vi "FCO_Open232.vi"(10 "port":u32, 11 "VISA resource name":refnum<visa-resource-name> caption="VISA资源名称") -> (0 "错误输出":errorcluster, 3 "status":bool)   [LabVIEW 2017]
uses:
  <vilib>/Instr/_visa.llb/VISA Configure Serial Port (Instr).vi
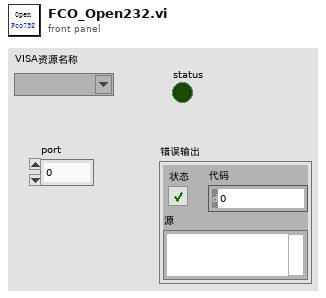
[diagram p1: front panel]
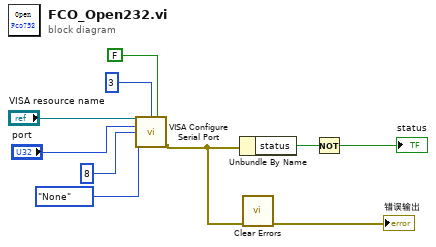
[diagram p0: block diagram]
diagram:
  n1 = call-poly "VISA Configure Serial Port"("VISA resource name"="VISA resource name", "termination char\n(0xA = '\\n' = LF)"=u8 3 ("termination char\n(0xA = '\\n' = LF)"), "Enable Termination\nChar (T)"=FALSE ("Enable Termination\nChar (T)"), "baud rate (9600)"="port", "data bits (8)"=u16 8, "parity (0:none)"=enum16{"None", "Odd", "Even", "Mark", "Space"}."None") -> ("error out"=w5:errorcluster)  [unwired: 4 in, 5 out]
  n2 = Unbundle By Name(w5) -> ("status"=w7:bool)
  n3 = call <vilib>:"Clear Errors.vi"("error in (no error)"=w5) -> ("error out"=→"错误输出":errorcluster)  [unwired: 5 in, 1 out]
  n4 = Not(x=w7) -> (.not. x?=→"status":bool)
